vi "SetFurniture.vi"(8 "error in (no error)":errorcluster, 10 "Furniture":refnum<class "Furniture.lvclass">[](array[class]), 11 "RoomA in":refnum<class "RoomA.lvclass">) -> (0 "error out":errorcluster, 3 "RoomA out":refnum<class "RoomA.lvclass">)   [LabVIEW 2019, in "RoomA.lvclass"]
uses:
  RoomA.lvclass
  Room.lvclass
  Furniture.lvclass
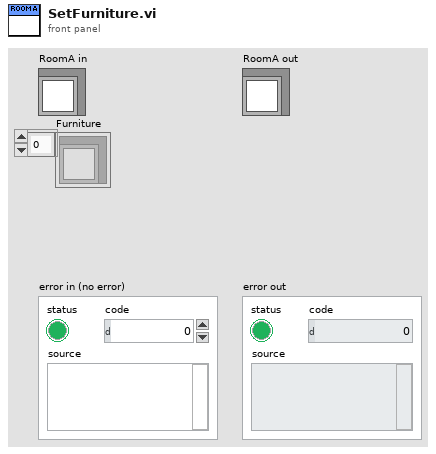
[diagram p1: front panel]
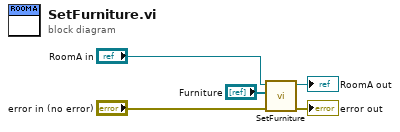
[diagram p0: block diagram]
diagram:
  n1 = call-parent "SetFurniture.vi"("error in (no error)"="error in (no error)", "Furniture"="Furniture", "Room in"="RoomA in") -> ("error out"=→"error out":errorcluster, "Room out"=→"RoomA out":refnum<class "RoomA.lvclass">)  [unwired: 7 in]
